vi "doc_delete_subtable_item.vi"(7 "subtables":string[](array[string]), 8 "error in (no error)":errorcluster, 9 "subkeys":string[](array[string]), 10 "Doc in":refnum<class "Doc.lvclass">) -> (0 "error out":errorcluster, 2 "Doc out":refnum<class "Doc.lvclass">, 4 "found?":bool)   [LabVIEW 2020, in "toml.lvclass"]
uses:
  toml.lvclass
  Doc/Doc.lvclass
  toml.lvclass/toml.ctl
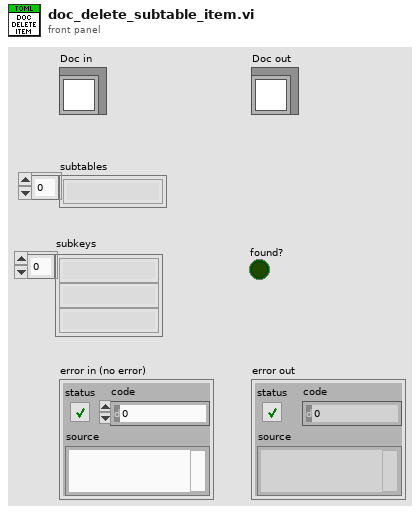
[diagram p1: front panel]
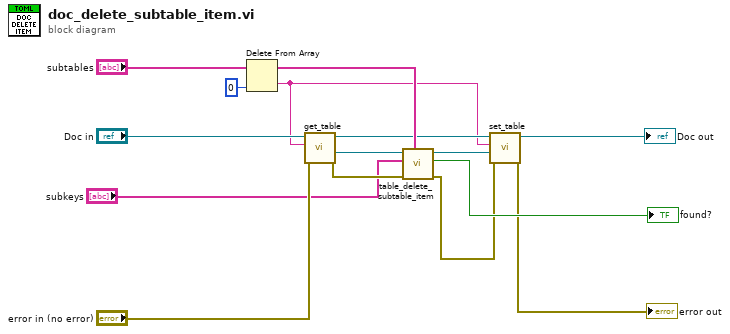
[diagram p0: block diagram]
diagram:
  n1 = Delete From Array(array="subtables", index=0) -> (deleted portion=w4:string, array with subset deleted=w15:string[])  [unwired: 1 in]
  n2 = call "get_table.vi"("error in (no error)"="error in (no error)", "table_name"=w4, "Doc in"="Doc in") -> ("error out"=w13:errorcluster, "Table"=w8:refnum<class "Table.lvclass">, "Doc out"=w6:refnum<class "Doc.lvclass">)  [unwired: 6 in]
  n3 = call "table_delete_subtable_item.vi"("subtables"=w15, "error in (no error)"=w13, "subkeys"="subkeys", "Table in"=w8) -> ("error out"=w2:errorcluster, "found?"=→"found?":bool, "Table out"=w3:refnum<class "Table.lvclass">)  [unwired: 5 in]
  n4 = call "set_table.vi"("error in (no error)"=w2, "Table"=w3, "table_name"=w4, "Doc in"=w6) -> ("error out"=→"error out":errorcluster, "Doc out"=→"Doc out":refnum<class "Doc.lvclass">)  [unwired: 6 in]
